vi "文件记录.vi"(9 "文件存储路径":path=path "C:/Users/dell/Desktop/record_chengming.txt", 10 "reference输入":refnum<vi>, 11 "Boolean输入":refnum<vi>) -> ()   [LabVIEW 2016]
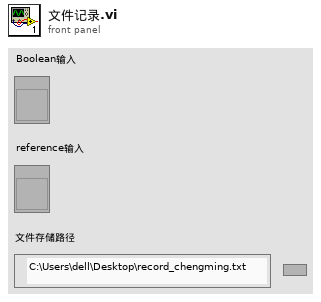
[diagram p1: front panel]
types:
  T1 = enum16{"open", "replace", "create", "open or create", "replace or create", "replace or create with confirmation"}
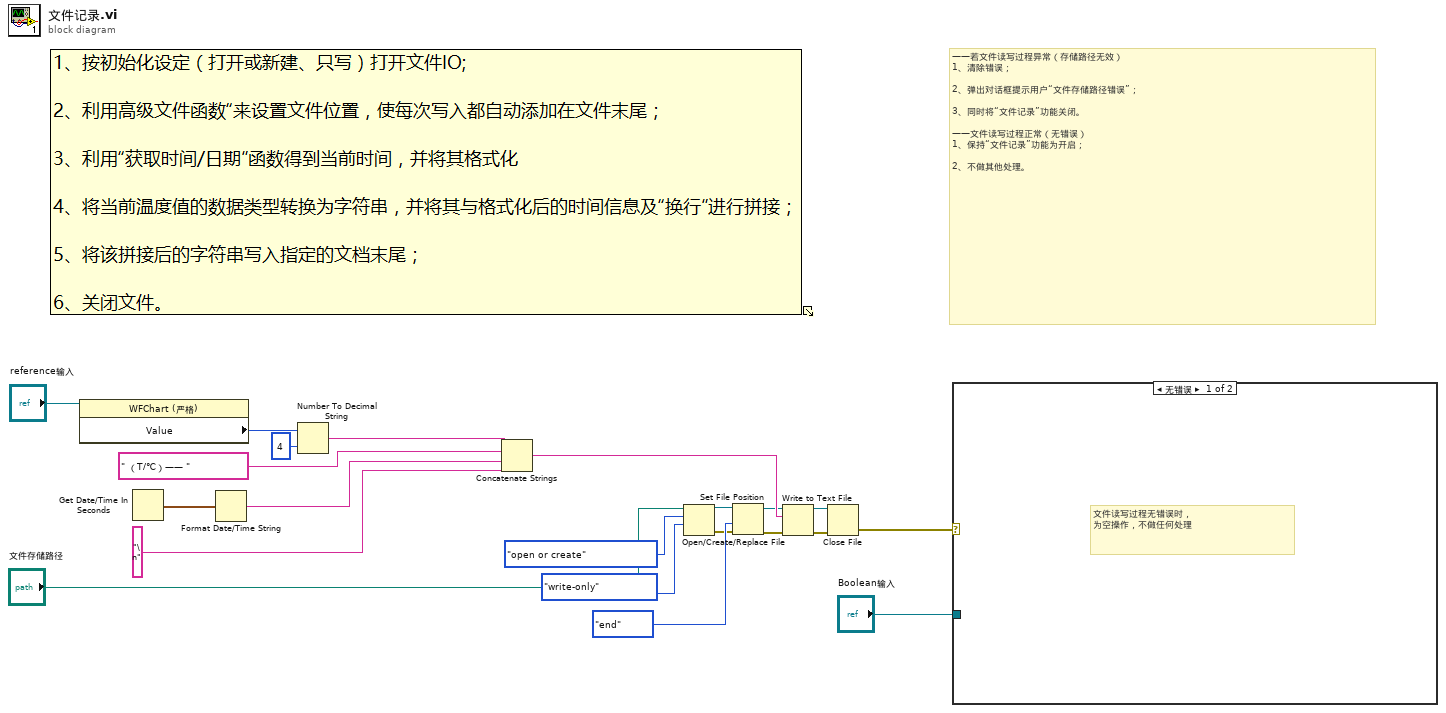
[diagram p0: block diagram]
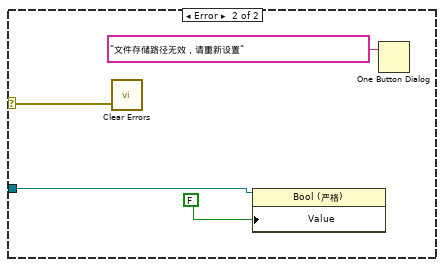
[diagram p2: hidden frame]
diagram:
  # "——若文件读写过程异常（存储路径无效）\n1、清除错误；\n\n2、弹出对话框提示用户“文件存储路径错误”；\n\n3、同时将“文件记录”功能关闭。\n\n——文件读写过程正常（无错误）\n1、保持“文件记录”功能为开启；\n\n2、不做其他处理。"
  n1 = property class="WFChart (严格)"(reference="reference输入") -> ("Value"=w20:i32)  [unwired: 1 in, 2 out]
  n2 = Get Date/Time In Seconds() -> (seconds since 1Jan1904=w9:timestamp)
  n3 = Format Date/Time String(seconds (now)=w9) -> (date/time string=w13:string)  [unwired: 2 in]
  n4 = Number To Decimal String(number=w20, width (-)=i16 4 ("宽度(-)")) -> (decimal integer string=w10:string)
  n5 = Concatenate Strings(w10, " （T/℃）—— " ("字符串"), w13, "\n" ("字符串")) -> (w17:string)
  n6 = Open/Create/Replace File(file path (use dialog)="文件存储路径", operation (0:open)=T1."open or create" ("操作(0:open)"), access (0:read/write)=enum16{"read/write", "read-only", "write-only"}."write-only" ("权限(0:read/write)")) -> (refnum out=w5:refnum<file>, error out=w4:errorcluster)  [unwired: 3 in, 1 out]
  n7 = Set File Position(refnum=w5, from (0:start)=enum16{"start", "end", "current"}."end" ("自（0:起始）"), error in=w4) -> (refnum out=w15:refnum<file>, error out=w16:errorcluster)  [unwired: 1 in]
  n8 = Write to Text File(file (use dialog)=w15, text=w17, error in=w16) -> (refnum out=w18:refnum<file>, error out=w19:errorcluster)  [unwired: 1 in, 1 out]
  n9 = Close File(refnum=w18, error in=w19) -> (error out=w3:errorcluster)  [unwired: 1 out]
  n10 = case shown="无错误" w3 {
    selector: w3 -> [_ w25]
    tunnel: "Boolean输入" -> [_ w22]
    frame No Error {
      # "文件读写过程无错误时，\n为空操作，不做任何处理"
    }
    frame Error {
      n11 = call <vilib>:"Clear Errors.vi"("error in (no error)"=w25) -> ()  [unwired: 5 in, 2 out]
      n12 = property class="Bool (严格)"(reference=w22, "Value"=FALSE) -> ()  [unwired: 1 in, 2 out]
      n13 = One Button Dialog(message="文件存储路径无效，请重新设置" ("消息")) -> ()  [unwired: 1 in, 1 out]
    }
  }
